vi "Change Access Scope of NI Lib.vi"(8 "Error In":errorcluster) -> (0 "Error Out":errorcluster)   [LabVIEW 2011, in "Generator.lvlib"]
doc: "This VI checks the access scope of a NI scripting library and changes it to public access for use in the generator."
uses:
  Generator.lvlib
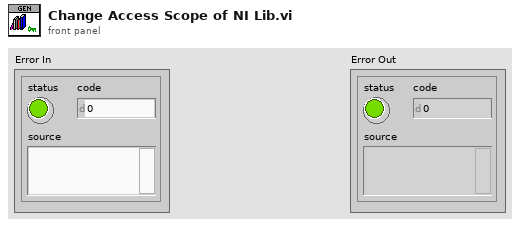
[diagram p1: front panel]
types:
  T1 = enum32{"invalid scope", "public", "private", "protected", "community"}
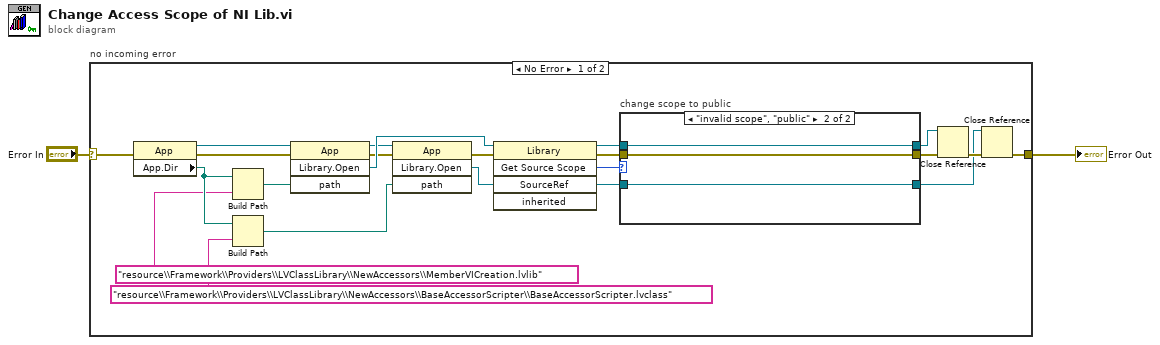
[diagram p0: block diagram]
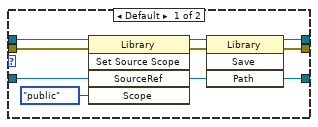
[diagram p2: hidden frame]
diagram:
  n1 = case "no incoming error" shown="No Error" "Error In" {
    selector: "Error In" -> [w23 w35]
    tunnel: [w3 w35] -> w1
    frame No Error {
      n2 = property class="App"(error in=w23) -> (reference out=w19:refnum<vi>, error out=w21:errorcluster, "App.Dir"=w15:path)  [unwired: 1 in]
      n3 = Build Path(base path=w15, name or relative path="resource\\Framework\\Providers\\LVClassLibrary\\NewAccessors\\MemberVICreation.lvlib") -> (appended path=w16:path)
      n4 = Build Path(base path=w15, name or relative path="resource\\Framework\\Providers\\LVClassLibrary\\NewAccessors\\BaseAccessorScripter\\BaseAccessorScripter.lvclass") -> (appended path=w13:path)
      n5 = invoke class="App" method="Library.Open"(reference=w19, error in=w21, "path"=w16) -> (reference out=w17:refnum<vi>, error out=w18:errorcluster, "Open Library"=w20:refnum<vi>)  [unwired: 1 in, 1 out]
      n6 = invoke class="App" method="Library.Open"(reference=w17, error in=w18, "path"=w13) -> (error out=w12:errorcluster, "Open Library"=w8:refnum<vi>)  [unwired: 1 in, 2 out]
      n7 = invoke class="Library" method="Get Source Scope"(reference=w20, error in=w12, "SourceRef"=w8) -> (reference out=w9:refnum<vi>, error out=w10:errorcluster, "GetSourceScope"=w11:T1)  [unwired: 2 in, 2 out]
      n8 = case "change scope to public" shown="\"invalid scope\", \"public\"" w11 {
        tunnel: w10 -> [w31 w34]
        tunnel: w9 -> [w30 w33]
        tunnel: w8 -> [w24 w32]
        tunnel: [w26 w34] -> w7
        tunnel: [w25 w33] -> w6
        tunnel: [w24 w32] -> w4
        frame Default {
          n9 = invoke class="Library" method="Set Source Scope"(reference=w30, error in=w31, "SourceRef"=w24, "Scope"=T1."public" ("scope")) -> (reference out=w27:refnum<vi>, error out=w28:errorcluster)  [unwired: 1 in, 3 out]
          n10 = invoke class="Library" method="Save"(reference=w27, error in=w28) -> (reference out=w25:refnum<vi>, error out=w26:errorcluster)  [unwired: 2 in, 2 out]
        }
        frame "invalid scope", "public" {
        }
      }
      n11 = Close Reference(reference=w6, error in (no error)=w7) -> (error out=w5:errorcluster)
      n12 = Close Reference(reference=w4, error in (no error)=w5) -> (error out=w3:errorcluster)
    }
    frame Error {
    }
  }
  "Error Out" <- w1
